vi "Set Tx UDP.vi"(8 "error in":errorcluster, 10 "Tx UDP configuration":T3(array[cluster]) {"tx_udp_setup"."NumOfSubVl" format="%.0b"; "tx_udp_setup"."NetSelect" items=["FDX_TX_FRAME_DLY_A", "FDX_TX_FRAME_DLY_B", "FDX_TX_FRAME_BOTH", "FDX_TX_FRAME_ONLY_A", "FDX_TX_FRAME_ONLY_B"]}, 11 "port ref":T4 format="%.0x") -> (0 "error out":errorcluster, 3 "port ref out":T4 format="%.0x")   [LabVIEW 2020, in "AIM ARINC 664 Scripting.lvlib"]
uses:
  AIM ARINC 664 Scripting.lvlib
  <vilib>/NI VeriStand/Custom Device API/Custom Device Item Ref.ctl
  <vilib>/NI/NI VeriStand Encoding and Decoding/Encoding.ctl
  Shared/frame_parameter_definition.ctl
  <vilib>/NI VeriStand/Custom Device API/Custom Device API.lvlib
  <vilib>/NI/NI VeriStand Encoding and Decoding/Encoding and Decoding.lvlib
  Import/AIM ARINC 664 Import.lvlib
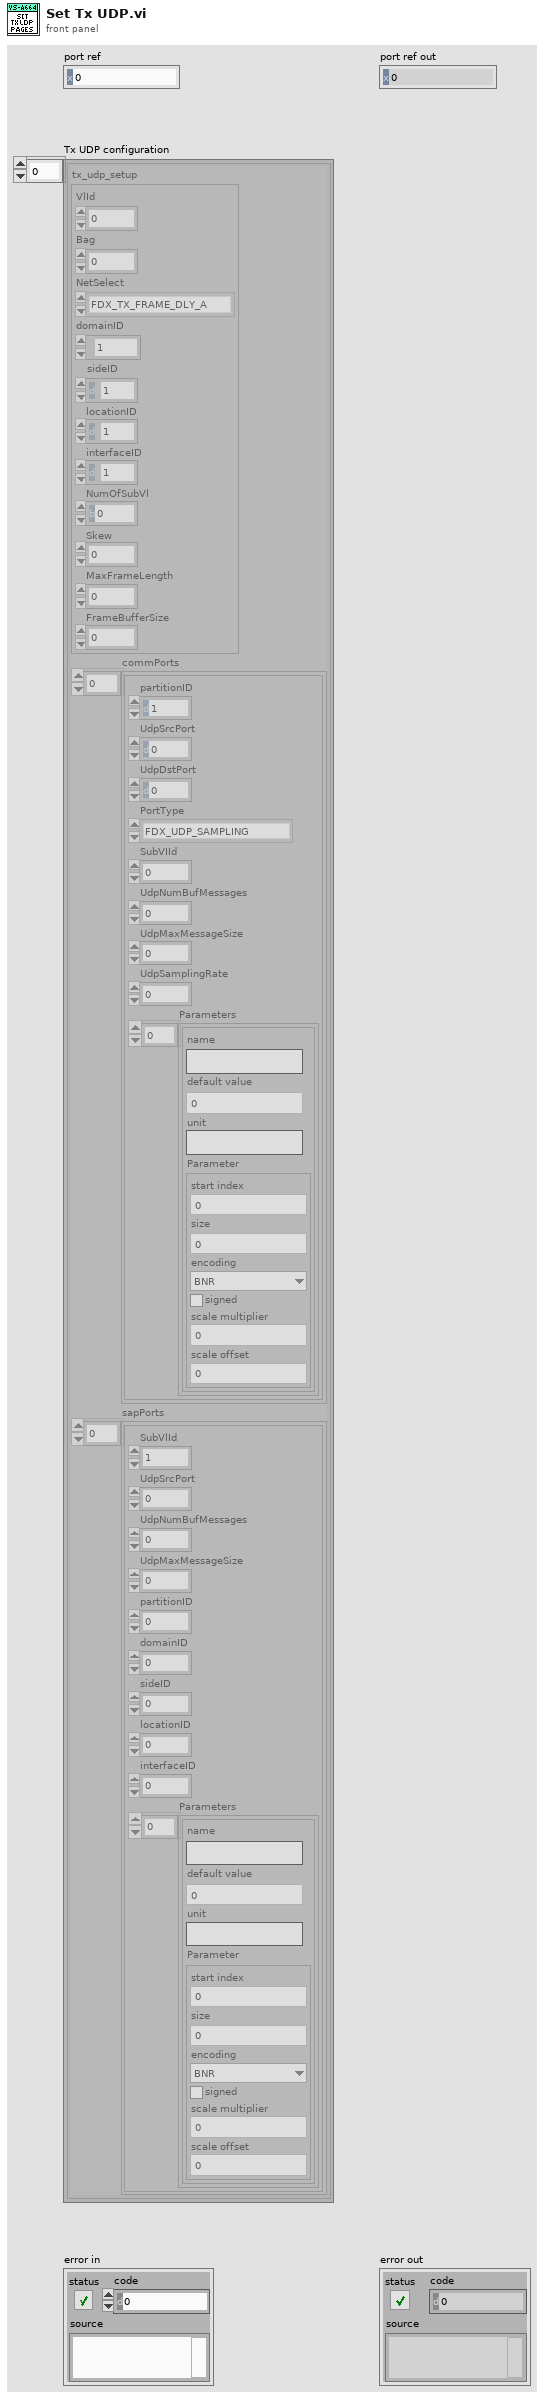
[diagram p1: front panel]
types:
  T1 = typedef "Encoding and Decoding.lvlib/Encoding.ctl" = enum16{"BNR", "BCD", "Discrete"}
  T2 = typedef "AIM ARINC 664 Import.lvlib/frame_parameter_definition.ctl" = cluster{"start index":i32, "size":i32, "encoding":T1, "signed":bool, "scale multiplier":dbl, "scale offset":dbl}
  T3 = cluster{"tx_udp_setup":cluster{"VlId":i32, "Bag":i32, "NetSelect":i32, "domainID":u8, "sideID":u8, "locationID":u8, "interfaceID":u8, "NumOfSubVl":u16, "Skew":u32, "MaxFrameLength":u32, "FrameBufferSize":u32}, "commPorts":cluster{"partitionID":u8, "UdpSrcPort":u16, "UdpDstPort":u16, "PortType":enum16{"FDX_UDP_SAMPLING", "FDX_UDP_QUEUING"}, "SubVIId":u32, "UdpNumBufMessages":u32, "UdpMaxMessageSize":u32, "UdpSamplingRate":u32, "Parameters":cluster{"name":string, "default value":dbl, "unit":string, "Parameter":cluster{"start index":i32, "size":i32, "encoding":T1, "signed":bool, "scale multiplier":dbl, "scale offset":dbl}}[]}[], "sapPorts":cluster{"SubVlId":u8, "UdpSrcPort":u16, "UdpNumBufMessages":u32, "UdpMaxMessageSize":u32, "partitionID":u8, "domainID":u8, "sideID":u8, "locationID":u8, "interfaceID":u8, "Parameters":cluster{"name":string, "default value":dbl, "unit":string, "Parameter":T2}[]}[]}[]
  T4 = typedef "Custom Device API.lvlib/Custom Device Item Ref.ctl" = u64
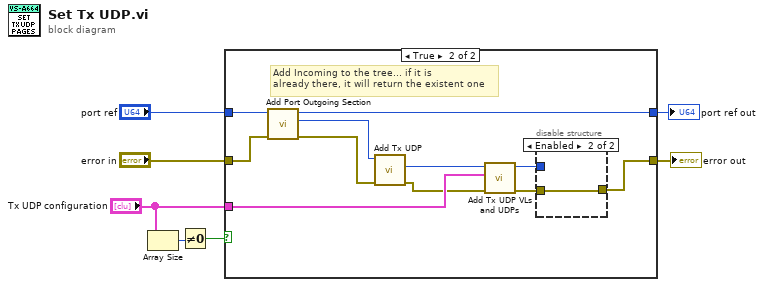
[diagram p0: block diagram]
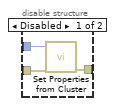
[diagram p3: hidden frame]
diagram:
  n1 = Array Size(array="Tx UDP configuration") -> (size(s)=w3:i32)
  n2 = Not Equal To 0?(x=w3) -> (x != 0?=w2:bool)
  n3 = case shown="True" w2 {
    tunnel: [w8 w20] -> w7
    tunnel: "error in" -> [w8 w19]
    tunnel: "port ref" -> [w9 w18]
    tunnel: [w9 w15] -> w4
    tunnel: "Tx UDP configuration" -> [_ w14]
    frame False {
      # "If Tx_Udp Cluster is empty, bypass this"
    }
    frame True {
      # "Add Incoming to the tree... if it is \nalready there, it will return the existent one"
      n4 = call "Add Port Outgoing Section.vi"("error in"=w19, "Port Ref"=w18) -> ("error out"=w17:errorcluster, "Port Outgoing Ref out"=w16:T4, "Port Ref out"=w15:T4)  [unwired: 7 in]
      n5 = call "Add Tx UDP.vi"("error in"=w17, "Port Outgoing Ref"=w16) -> ("error out"=w12:errorcluster, "Section Ptr"=w13:T4)  [unwired: 7 in, 1 out]
      n6 = call "Add Tx UDP VLs and UDPs.vi"("error in (no error)"=w12, "Tx_UDP"=w14, "Section Ref in in"=w13) -> ("error out"=w11:errorcluster, "Section Ref out"=w10:T4)  [unwired: 7 in]
      n7 = disable-structure shown="Enabled" {
        disable-tunnel: [w23 w24] -> w20
        disable-tunnel: w11 -> [w22 w24]
        disable-tunnel: w10 -> [w21 _]
        frame Disabled {
          n8 = call "Set Properties from Cluster.vi"("error in"=w22, "item ref in"=w21) -> ("error out"=w23:errorcluster)  [unwired: 8 in, 1 out]
        }
        frame Enabled {
        }
      }
    }
  }
  "error out" <- w7
  "port ref out" <- w4
